vi "Motors Sub 03.vi"(7 "Cluster":T1, 8 "error in":errorcluster, 11 "VISA in":refnum<visa-resource-name>) -> (0 "error out":errorcluster, 3 "VISA out":refnum<visa-resource-name>)   [LabVIEW 2010]
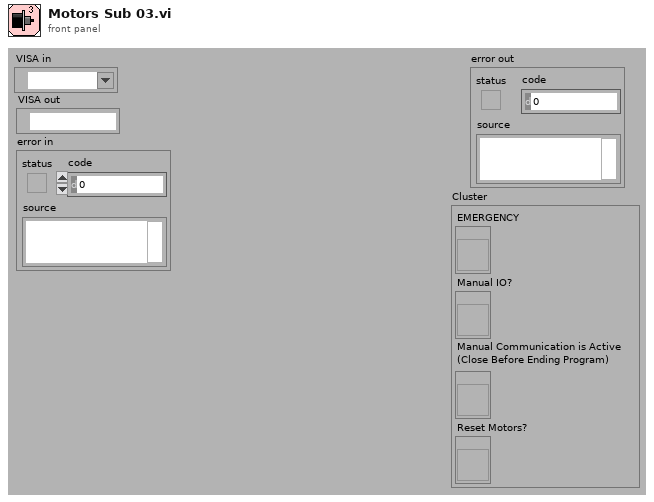
[diagram p1: front panel]
types:
  T1 = cluster{"EMERGENCY":refnum<vi>, "Manual IO?":refnum<vi>, "Manual Communication is Active\n(Close Before Ending Program)":refnum<vi>, "Reset Motors?":refnum<vi>}
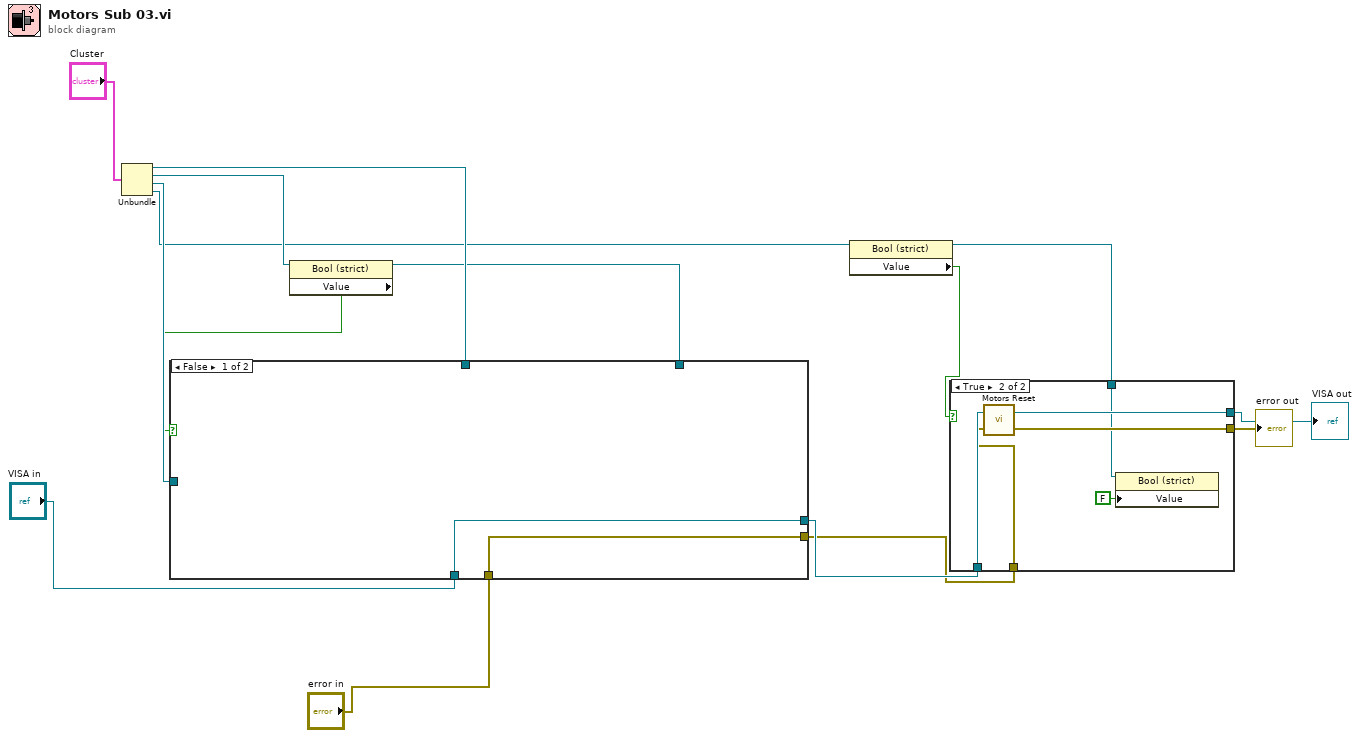
[diagram p0: block diagram]
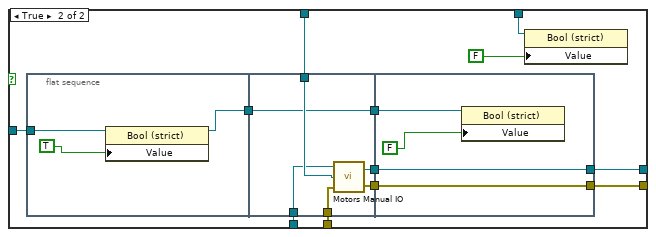
[diagram p3: hidden frame]
diagram:
  n1 = Unbundle("Cluster") -> ("EMERGENCY"=w12:refnum<vi>, "Manual IO?"=w9:refnum<vi>, "Manual Communication is Active\n(Close Before Ending Program)"=w11:refnum<vi>, "Reset Motors?"=w7:refnum<vi>)
  n2 = property on="Property Node" class="Bool (strict)"(reference=w9) -> (reference out=w8:refnum<vi>, "Value"=w10:bool)  [unwired: 1 in, 1 out]
  n3 = case shown="False" w10 {
    tunnel: [w16 w29] -> w13
    tunnel: [w17 w19] -> w14
    tunnel: w12 -> [_ w26]
    tunnel: w11 -> [_ w25]
    tunnel: w8 -> [_ w21]
    tunnel: "VISA in" -> [w17 w20]
    tunnel: "error in" -> [w16 w18]
    frame False {
    }
    frame True {
      n4 = flat-sequence {
        tunnel: w25 -> [w31]
        tunnel: [w30] -> w23
        tunnel: [w38] -> w28
        tunnel: [w37] -> w27
        tunnel: w26 -> [w36]
        tunnel: [w35] -> w24
        tunnel: w23 -> [w35]
        tunnel: w20 -> [w34]
        tunnel: w18 -> [w33]
        tunnel: [w41] -> w19
        tunnel: [w42] -> w29
        tunnel: w28 -> [w42]
        tunnel: w27 -> [w41]
        tunnel: w24 -> [w39]
        frame #0 {
          n5 = property on="Property Node" class="Bool (strict)"(reference=w31, "Value"=TRUE ("Manual Communication is Active\n(Close Before Ending Program) 2")) -> (reference out=w30:refnum<vi>)  [unwired: 1 in, 1 out]
        }
        frame #1 {
          n6 = call "Motors Manual IO.vi"("error in"=w33, "Emergency Stop Reference"=w36, "VISA in"=w34) -> ("error out"=w38:errorcluster, "VISA out"=w37:refnum<visa-resource-name>)
        }
        frame #2 {
          n7 = property on="Property Node" class="Bool (strict)"(reference=w39, "Value"=FALSE ("Manual Communication is Active\n(Close Before Ending Program)")) -> ()  [unwired: 1 in, 2 out]
        }
      }
      n8 = property on="Property Node" class="Bool (strict)"(reference=w21, "Value"=FALSE) -> ()  [unwired: 1 in, 2 out]
    }
  }
  n9 = property on="Property Node" class="Bool (strict)"(reference=w7) -> (reference out=w5:refnum<vi>, "Value"=w6:bool)  [unwired: 1 in, 1 out]
  n10 = case shown="True" w6 {
    tunnel: [w43 w50] -> w2
    tunnel: [w44 w49] -> w4
    tunnel: w14 -> [w44 w48]
    tunnel: w13 -> [w43 w47]
    tunnel: w5 -> [_ w45]
    frame False {
    }
    frame True {
      n11 = call "Motors Reset.vi"("error in"=w47, "VISA in"=w48) -> ("error out"=w50:errorcluster, "VISA out"=w49:refnum<visa-resource-name>)
      n12 = property on="Property Node" class="Bool (strict)"(reference=w45, "Value"=FALSE) -> ()  [unwired: 1 in, 2 out]
    }
  }
  "VISA out" <- w4
  "error out" <- w2
